vi "LightOn.vi"(1 "Turns off when...":bool) -> (0 "Light Indicator":bool)   [LabVIEW 2018]
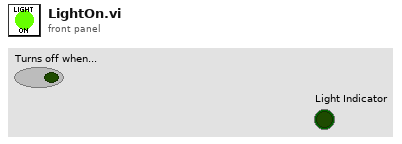
[diagram p1: front panel]
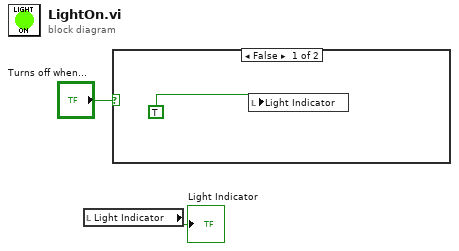
[diagram p0: block diagram]
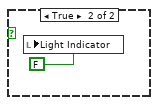
[diagram p2: hidden frame]
diagram:
  n1 = local read "Light Indicator"() -> (→"Light Indicator":bool)
  n2 = case shown="False" "Turns off when..." {
    frame False {
      n3 = local write "Light Indicator"(TRUE) -> ()
    }
    frame True {
      n4 = local write "Light Indicator"(FALSE) -> ()
    }
  }
